vi "Previous Station Check.vi"() -> ()   [LabVIEW 2020]
uses:
  Control Button/RPT.ctl
  <vilib>/Utility/error.llb/whitespace.ctl
  <vilib>/addons/database/Connection.llb/DB Tools Open Connec (String).vi
  Galobal variable_TI.vi
  <vilib>/Utility/file.llb/Read Delimited Spreadsheet (string).vi
  Project Setup/Globle Variable/GR_Servo.vi
  <vilib>/Utility/file.llb/Write Delimited Spreadsheet (string).vi
  <vilib>/addons/database/NI_Database_API.lvlib
panel:
  out "error out 5":errorcluster
  out "array 2":string[][](array[string])
  out "error out 4":errorcluster
  out "size(s)":i32
  out "error out 3":errorcluster
  out "array":string[][](array[string])
  out "error out 2":errorcluster
  out "error out":errorcluster
  in  "stop":bool
  in  "RPT":T1
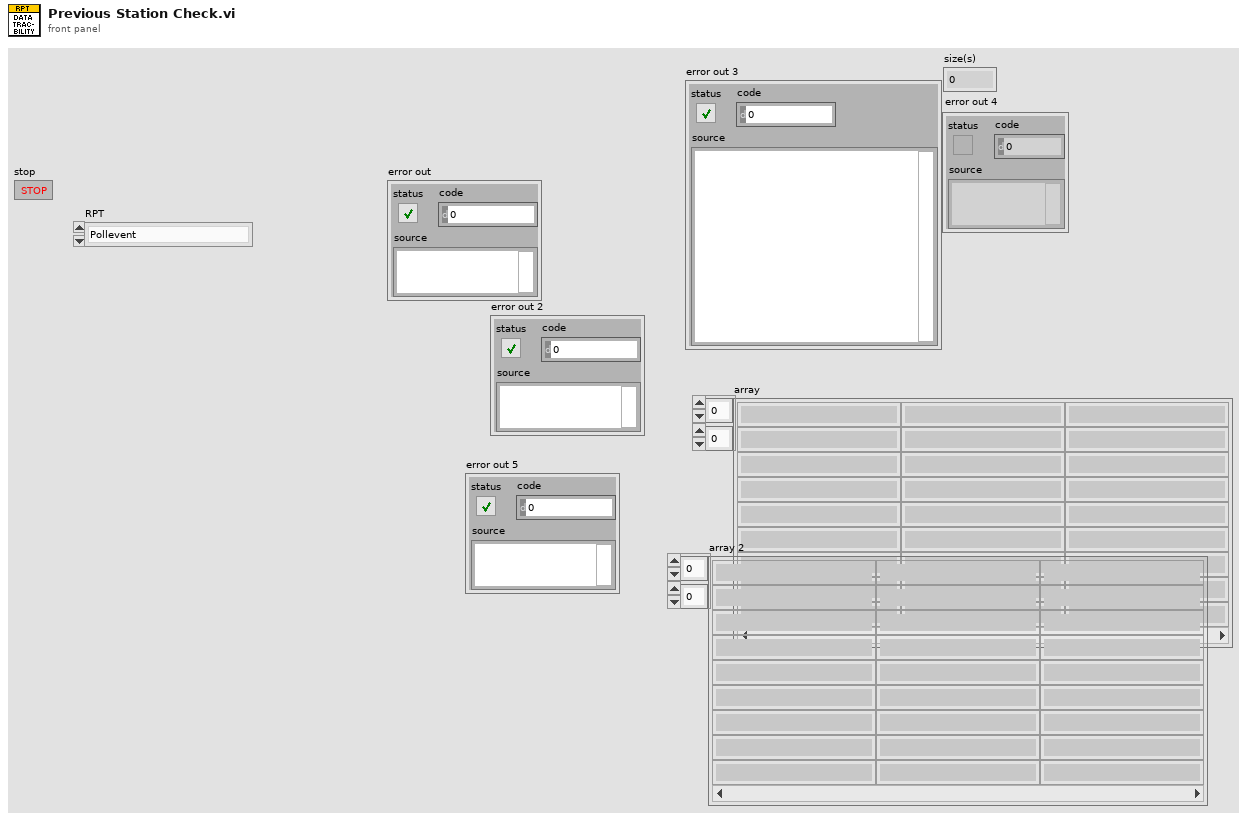
[diagram p1: front panel]
types:
  T1 = typedef "RPT.ctl" = enum16{"Pollevent", "Read", "Write", "Delete"}
  T2 = cluster{"Stn Name":string, "date":string, "time":string, "Operator id":string, "Shift":string, "Error Code":string, "Fail count":string, "Rework":string, "NA":string, "Tested":string}
  T3 = typedef "NI_Database_API.lvlib/Conn ObjectReference.ctl" = refnum<k1>
  T4 = enum16{"open", "replace", "create", "open or create", "replace or create", "replace or create with confirmation"}
  T5 = typedef "whitespace.ctl" = u16
  T6 = cluster{"Report data[0]":string, "Report data[1]":string, "Report data[2]":string, "Report data[3]":string, "Report data[4]":string, "Report data[5]":string, "Report data[6]":string, "Report data[7]":string, "Report data[8]":string, "Report data[9]":string, "Report data[10]":string, "Report data[11]":string, "Report data[12]":string, "Report data[13]":string, "Report data[14]":string, "Report data[15]":string}
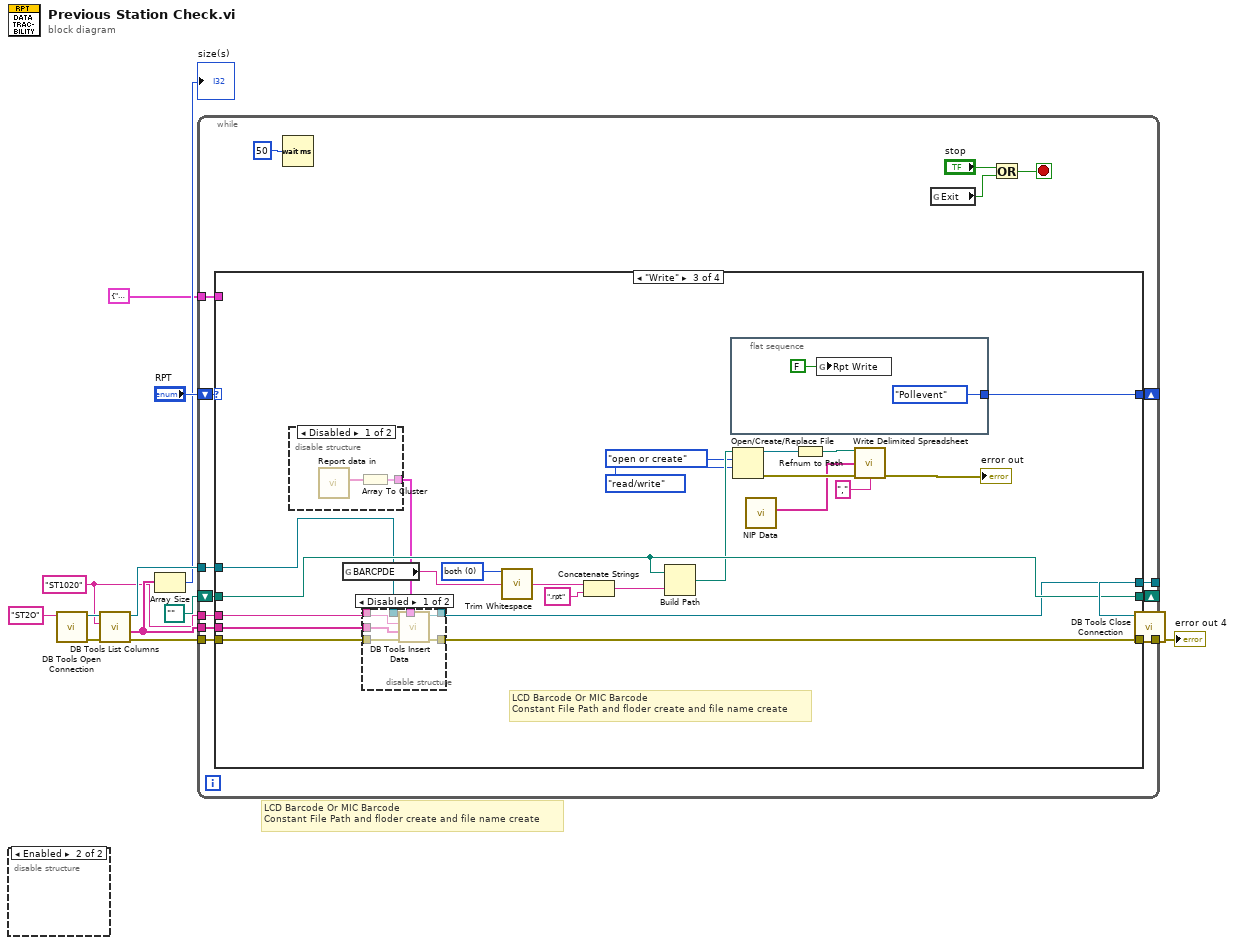
[diagram p0: block diagram]
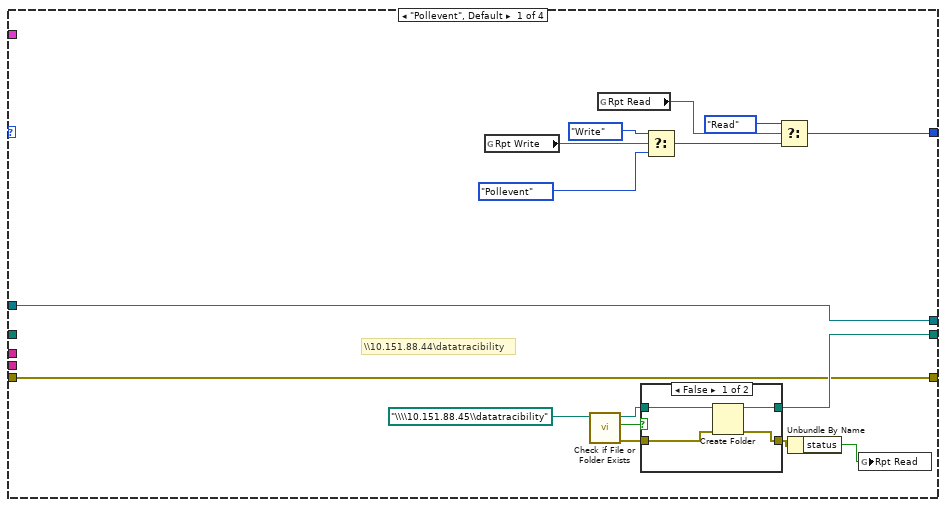
[diagram p2: hidden frame]
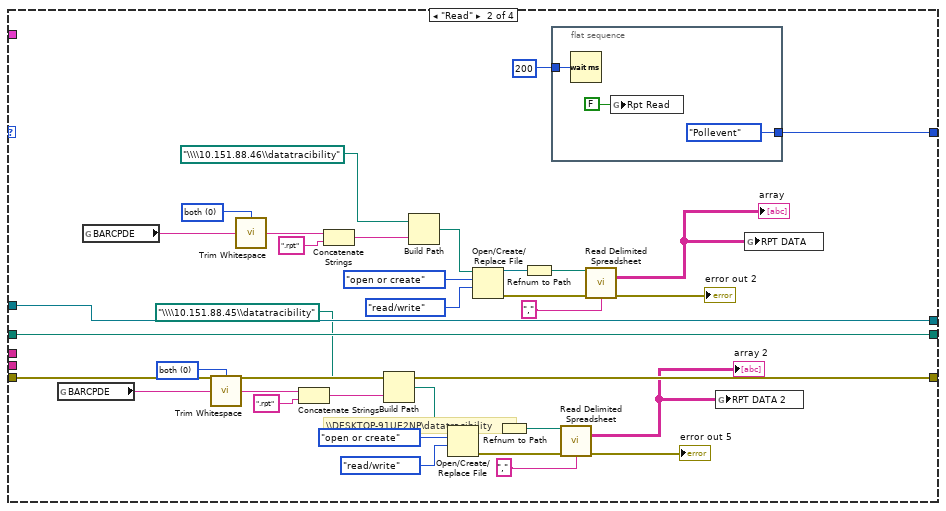
[diagram p4: hidden frame]
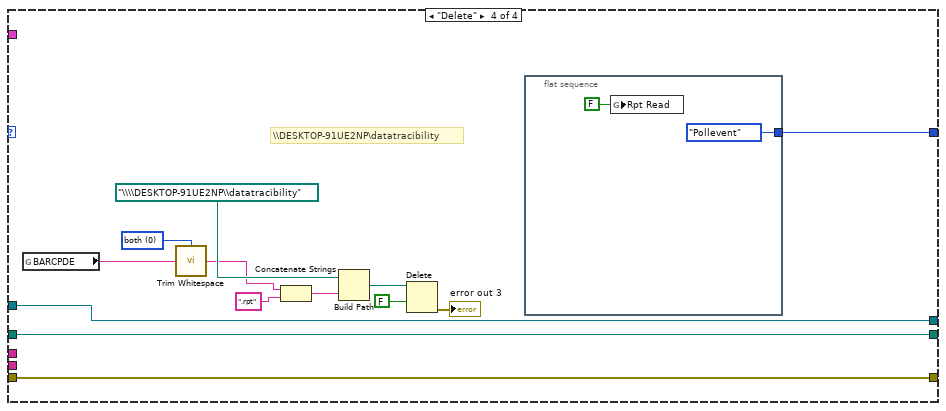
[diagram p7: hidden frame]
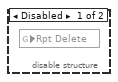
[diagram p8: hidden frame]
diagram:
  w6 = "ST1020" ("table")
  # "LCD Barcode Or MIC Barcode \nConstant File Path and floder create and file name create"
  n1 = disable-structure shown="Enabled" {
    frame Disabled {
      n2 = global read "Galobal variable_TI.vi" "Rpt Delete"() -> ()  [unwired: 1 in]
    }
    frame Enabled {
    }
  }
  n3 = call-poly <vilib>:"DB Tools Open Connection.vi"("connection information"="ST2O" ("string")) -> ("error out"=w11:errorcluster, "connection reference"=w12:T3)  [unwired: 7 in]
  n4 = call <vilib>:"DB Tools List Columns.vi"("error in (no error)"=w11, "table"=w6, "connection reference"=w12) -> ("error out"=w8:errorcluster, "columns"=w7:string[], "connection reference out"=w9:T3)  [unwired: 1 in, 1 out]
  n5 = Array Size(array=w7) -> (size(s)=→"size(s)":i32)
  n6 = while {
    shift-right: [w29] -> _
    shift-left: "RPT" -> [w28]
    shift-right: [w27] -> _
    shift-left: path "" ("created path") -> [w26]
    tunnel: w9 -> [w21]
    tunnel: w8 -> [w20]
    tunnel: w7 -> [w19]
    tunnel: w6 -> [w18]
    tunnel: [w17] -> w5
    tunnel: [w16] -> w4
    tunnel: T2 {"Stn Name"="", "date"="", "time"="", "Operator id"="", "Shift"="", "Error Code"="", "Fail count"="", "Rework"="", "NA"="", "Tested"=""} ("Write Data") -> [w15]
    stop <- w22 stop-if-true
    n7 = case shown="\"Write\"" w28 {
      tunnel: [w39 w86 w112 w136] -> w29
      tunnel: [w34 w80 w109 w133] -> w27
      tunnel: w26 -> [_ w80 w109 w133]
      tunnel: w21 -> [w33 w77 w102 w129]
      tunnel: w20 -> [w32 w76 w101 w128]
      tunnel: w19 -> [_ _ w100 _]
      tunnel: w18 -> [_ _ w99 _]
      tunnel: [w33 w77 w98 w129] -> w17
      tunnel: [w32 w76 w97 w128] -> w16
      tunnel: w15 -> [_ _ _ _]
      frame "Pollevent", Default {
        # "\\\\10.151.88.44\\datatracibility"
        n8 = global read "Galobal variable_TI.vi" "Rpt Write"() -> (w43:bool)
        n9 = call <vilib>:"Check if File or Folder Exists.vi"("path"=path "\\\\10.151.88.45\\datatracibility" ("base path")) -> ("error out"=w35:errorcluster, "file or folder exists?"=w37:bool, "dup path"=w36:path)  [unwired: 8 in]
        n10 = global read "Galobal variable_TI.vi" "Rpt Read"() -> (w44:bool)
        n11 = case shown="False" w37 {
          tunnel: w36 -> [w49 w51]
          tunnel: w35 -> [w48 w50]
          tunnel: [w47 w51] -> w34
          tunnel: [w46 w50] -> w31
          frame False {
            n12 = Create Folder(path (use dialog)=w49, error in=w48) -> (created path=w47:path, error out=w46:errorcluster)  [unwired: 1 in, 1 out]
          }
          frame True {
          }
        }
        n13 = Select(t=RPT."Write" ("RPT"), s=w43, f=RPT."Pollevent" ("RPT")) -> (s? t:f=w41:T1)
        n14 = Select(t=RPT."Read" ("RPT"), s=w44, f=w41) -> (s? t:f=w39:T1)
        n15 = Unbundle By Name(w31) -> ("status"=w30:bool)
        n16 = global write "Galobal variable_TI.vi" "Rpt Read"(w30) -> ()
      }
      frame "Read" {
        w59 = T5 0 items=["both", "start of string", "end of string"] ("location (both)")
        w74 = T5 0 items=["both", "start of string", "end of string"] ("location (both)")
        # "\\\\DESKTOP-91UE2NP\\datatracibility"
        n17 = global read "Galobal variable_TI.vi" "BARCPDE"() -> (w58:string)
        n18 = global read "Galobal variable_TI.vi" "BARCPDE"() -> (w75:string)
        n19 = call <vilib>:"Trim Whitespace.vi"("string"=w58, "location (both)"=w59) -> ("trimmed string"=w60:string)
        n20 = call <vilib>:"Trim Whitespace.vi"("string"=w75, "location (both)"=w74) -> ("trimmed string"=w73:string)
        n21 = Concatenate Strings(w60, ".rpt" ("string")) -> (w53:string)
        n22 = Concatenate Strings(w73, ".rpt" ("string")) -> (w84:string)
        n23 = Build Path(base path=path "\\\\10.151.88.45\\datatracibility", name or relative path=w53) -> (appended path=w54:path)
        n24 = Build Path(base path=path "\\\\10.151.88.46\\datatracibility", name or relative path=w84) -> (appended path=w83:path)
        n25 = Open/Create/Replace File(file path (use dialog)=w54, operation (0:open)=T4."open or create", access (0:read/write)=enum16{"read/write", "read-only", "write-only"}."read/write") -> (refnum out=w62:refnum<file>, error out=w57:errorcluster)  [unwired: 3 in, 1 out]
        n26 = Open/Create/Replace File(file path (use dialog)=w83, operation (0:open)=T4."open or create", access (0:read/write)=enum16{"read/write", "read-only", "write-only"}."read/write") -> (refnum out=w71:refnum<file>, error out=w79:errorcluster)  [unwired: 3 in, 1 out]
        n27 = Refnum to Path(1:w62) -> (0:w63:path)
        n28 = Refnum to Path(1:w71) -> (0:w70:path)
        n29 = flat-sequence {
          tunnel: [RPT."Pollevent" ("RPT")] -> w86
          tunnel: u32 200 ("milliseconds to wait") -> [w87]
          frame #0 {
            n30 = Wait (ms)(milliseconds to wait=w87) -> ()  [unwired: 1 out]
            n31 = global write "Galobal variable_TI.vi" "Rpt Read"(FALSE ("Rpt Read")) -> ()
          }
        }
        n32 = call-poly <vilib>:"Read Delimited Spreadsheet.vi"("file path (dialog if empty)"=w63, "error in (no error)"=w57, "delimiter (\\t)"="," ("delimiter (\\t)")) -> ("all rows"=w65:string[][], "error out"=→"error out 5":errorcluster)  [unwired: 7 in, 4 out]
        "array 2" <- w65
        n33 = call-poly <vilib>:"Read Delimited Spreadsheet.vi"("file path (dialog if empty)"=w70, "error in (no error)"=w79, "delimiter (\\t)"="," ("delimiter (\\t)")) -> ("all rows"=w68:string[][], "error out"=→"error out 2":errorcluster)  [unwired: 7 in, 4 out]
        "array" <- w68
        n34 = global write "GR_Servo.vi" "RPT DATA 2"(w65) -> ()
        n35 = global write "GR_Servo.vi" "RPT DATA"(w68) -> ()
      }
      frame "Write" {
        w93 = T5 0 items=["both", "start of string", "end of string"] ("location (both)")
        # "LCD Barcode Or MIC Barcode \nConstant File Path and floder create and file name create"
        n36 = disable-structure shown="Disabled" {
          disable-tunnel: [w113 _] -> w96
          frame Disabled {
            n37 = call "Report data in.vi"() -> ("Report data"=w114:string[])  [unwired: 11 in]
            n38 = Array To Cluster(array=w114) -> (cluster=w113:T6)
          }
          frame Enabled {
          }
        }
        n39 = global read "Galobal variable_TI.vi" "BARCPDE"() -> (w95:string)
        n40 = disable-structure shown="Disabled" {
          disable-tunnel: w102 -> [w121 _]
          disable-tunnel: w101 -> [w120 _]
          disable-tunnel: w100 -> [w119 _]
          disable-tunnel: w99 -> [w118 _]
          disable-tunnel: [w117 _] -> w98
          disable-tunnel: [w116 _] -> w97
          disable-tunnel: w96 -> [w115 _]
          frame Disabled {
            n41 = call <vilib>:"DB Tools Insert Data.vi"("data"=w115, "error in (no error)"=w120, "columns"=w119, "table"=w118, "connection reference"=w121) -> ("error out"=w116:errorcluster, "connection reference out"=w117:T3)  [unwired: 5 in]
          }
          frame Enabled {
          }
        }
        n42 = call <vilib>:"Trim Whitespace.vi"("string"=w95, "location (both)"=w93) -> ("trimmed string"=w94:string)
        n43 = Concatenate Strings(w94, ".rpt" ("string")) -> (w110:string)
        n44 = Build Path(base path=w109, name or relative path=w110) -> (appended path=w108:path)
        n45 = flat-sequence {
          tunnel: [RPT."Pollevent" ("RPT")] -> w112
          frame #0 {
            n46 = global write "Galobal variable_TI.vi" "Rpt Write"(FALSE ("Rpt Read")) -> ()
          }
        }
        n47 = Open/Create/Replace File(file path (use dialog)=w108, operation (0:open)=T4."open or create", access (0:read/write)=enum16{"read/write", "read-only", "write-only"}."read/write") -> (refnum out=w105:refnum<file>, error out=w103:errorcluster)  [unwired: 3 in, 1 out]
        n48 = call "NIP Data.vi"() -> ("Data"=w91:string[])  [unwired: 11 in]
        n49 = Refnum to Path(1:w105) -> (0:w104:path)
        n50 = call-poly <vilib>:"Write Delimited Spreadsheet.vi"("file path (dialog if empty)"=w104, "1D data"=w91, "error in (no error)"=w103, "delimiter (\\t)"="," ("delimiter (\\t)")) -> ("error out"=→"error out":errorcluster)  [unwired: 10 in, 1 out]
      }
      frame "Delete" {
        w126 = T5 0 items=["both", "start of string", "end of string"] ("location (both)")
        # "\\\\DESKTOP-91UE2NP\\datatracibility"
        n51 = global read "Galobal variable_TI.vi" "BARCPDE"() -> (w125:string)
        n52 = call <vilib>:"Trim Whitespace.vi"("string"=w125, "location (both)"=w126) -> ("trimmed string"=w124:string)
        n53 = Concatenate Strings(w124, ".rpt" ("string")) -> (w134:string)
        n54 = Build Path(base path=path "\\\\DESKTOP-91UE2NP\\datatracibility", name or relative path=w134) -> (appended path=w132:path)
        n55 = Delete(path (use dialog)=w132, confirm (F)=FALSE) -> (error out=→"error out 3":errorcluster)  [unwired: 3 in, 2 out]
        n56 = flat-sequence {
          tunnel: [RPT."Pollevent" ("RPT")] -> w136
          frame #0 {
            n57 = global write "Galobal variable_TI.vi" "Rpt Read"(FALSE ("Rpt Read")) -> ()
          }
        }
      }
    }
    n58 = Wait (ms)(milliseconds to wait=u32 50) -> ()  [unwired: 1 out]
    n59 = global read "Galobal variable_TI.vi" "Exit"() -> (w24:bool)
    n60 = Or(x="stop", y=w24) -> (x .or. y?=w22:bool)
  }
  n61 = call <vilib>:"DB Tools Close Connection.vi"("error in (no error)"=w4, "connection reference"=w5) -> ("error out"=→"error out 4":errorcluster)  [unwired: 5 in]
